vi "Set Voltage.vi"(8 "error in (no error)":errorcluster, 10 "V":dbl, 11 "SR3XXX HVPS in":refnum<class "SR3XXX HVPS.lvclass">) -> (0 "error out":errorcluster, 3 "SR3XXX HVPS out":refnum<class "SR3XXX HVPS.lvclass">)   [LabVIEW 2014, in "SR3XXX HVPS.lvclass"]
uses:
  SR3XXX HVPS.lvclass
  reusable/Session APIs/Serial/Typedefs/Session Handle.ctl
  reusable/Session APIs/Serial/Serial Session.lvclass
  Base/Session HVPS.lvclass/Session HVPS.ctl
  Base/Read hSession.vi
  Base/Write Vsp.vi
  reusable/Session APIs/Serial/Public/Asynchronous Write.vi
  <userlib>/_Session Fwk/Session - Root.lvclass
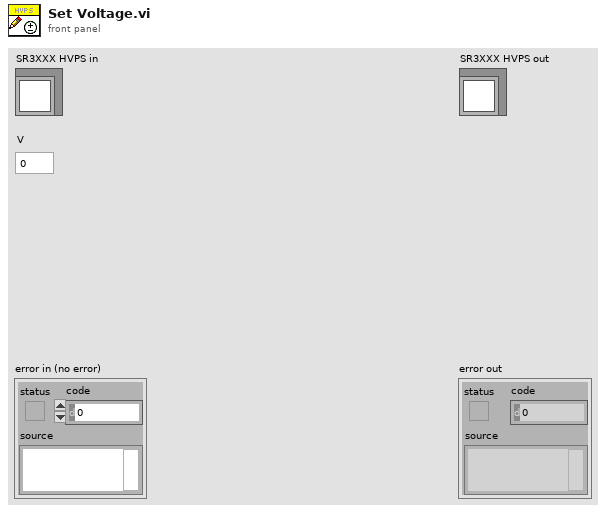
[diagram p1: front panel]
types:
  T1 = typedef "Serial Session.lvclass/Session Handle.ctl" = refnum<data-value>
  T2 = typedef "Session - Root.lvclass/Session Handle.ctl" = refnum<data-value>
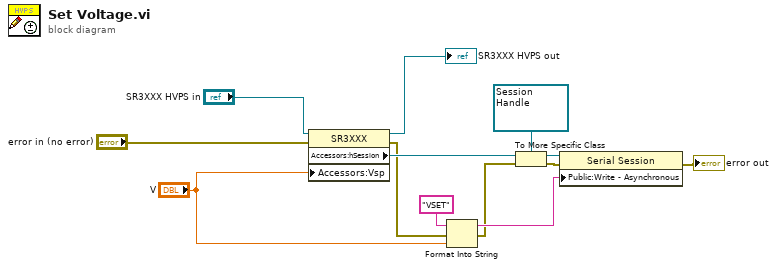
[diagram p0: block diagram]
diagram:
  n1 = property class="SR3XXX"(reference="SR3XXX HVPS in", error in="error in (no error)", "Accessors:Vsp"="V") -> (reference out=→"SR3XXX HVPS out":refnum<class "SR3XXX HVPS.lvclass">, error out=w2:errorcluster, "Accessors:hSession"=w11:T2)
  n2 = Format Into String(initial string="VSET", error in=w2, "V") -> (resulting string=w6:string, error out=w1:errorcluster)  [unwired: 1 in]
  n3 = To More Specific Class(target class=T1 refnum ("Session Handle"), reference=w11, error in=w1) -> (specific class reference=w7:T1, error out=w12:errorcluster)
  n4 = property class="Serial Session"(reference=w7, error in=w12, "Public:Write - Asynchronous"=w6) -> (error out=→"error out":errorcluster)  [unwired: 1 out]
